vi "Read Sub Panel Products.vi"(8 "error in (no error)":errorcluster, 11 "Cafe in":refnum<class "Cafe.lvclass">) -> (0 "error out":errorcluster, 2 "Sub Panel Products":refnum<vi>, 3 "Cafe out":refnum<class "Cafe.lvclass">)   [LabVIEW 2020, in "Cafe.lvlib" / "Cafe.lvclass"]
uses:
  Cafe.lvclass
  Cafe.lvclass/Cafe.ctl
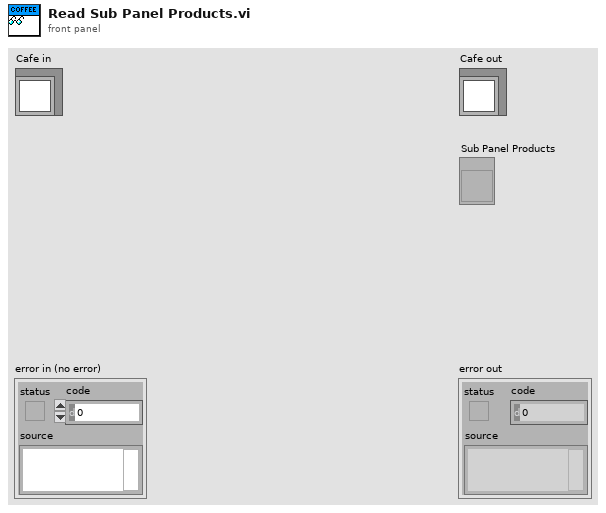
[diagram p1: front panel]
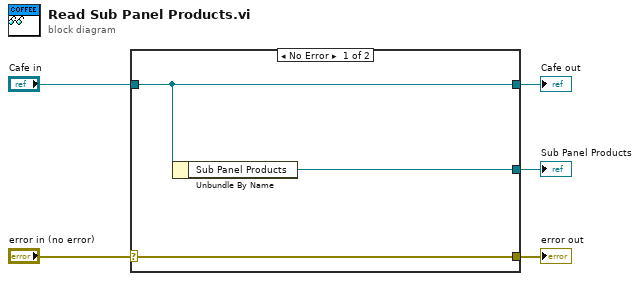
[diagram p0: block diagram]
diagram:
  n1 = case shown="No Error" "error in (no error)" {
    selector: "error in (no error)" -> [w8 w9]
    tunnel: [w8 w9] -> w4
    tunnel: [w7 w10] -> w2
    tunnel: "Cafe in" -> [w7 w10]
    tunnel: [w6 _] -> w1
    frame No Error {
      n2 = Unbundle By Name(w7) -> ("Sub Panel Products"=w6:refnum<vi>)
    }
    frame Error {
    }
  }
  "error out" <- w4
  "Cafe out" <- w2
  "Sub Panel Products" <- w1
